vi "ARITHMATIC_OPERATIONS.vi"() -> ()   [LabVIEW 2020]
panel:
  out "DEVISION":dbl
  out "MULTIPLICATION5":dbl
  out "SUBSTIRACTION":dbl
  in  "?":dbl
  out "ADDITION":dbl
  in  "NUMBER 1":dbl
  # "NUMBER 2"
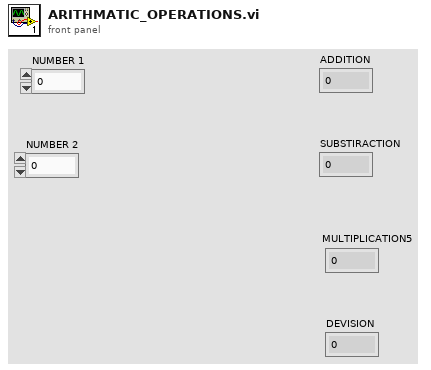
[diagram p1: front panel]
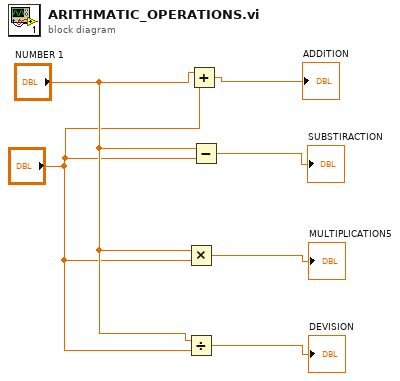
[diagram p0: block diagram]
diagram:
  n1 = Multiply(x="NUMBER 1", y="?") -> (x*y=→"MULTIPLICATION5":dbl)
  n2 = Divide(x="NUMBER 1", y="?") -> (x/y=→"DEVISION":dbl)
  n3 = Add(x="NUMBER 1", y="?") -> (x+y=→"ADDITION":dbl)
  n4 = Subtract(x="NUMBER 1", y="?") -> (x-y=→"SUBSTIRACTION":dbl)
